vi "Get ChildType.vi"(8 "error in (no error)":errorcluster, 11 "LVArrayType.lvclass in":refnum<class "LVArrayType.lvclass">) -> (0 "error out":errorcluster, 2 "ChildType":refnum<class "LVType.lvclass">, 3 "LVArrayType.lvclass out":refnum<class "LVArrayType.lvclass">)   [LabVIEW 2020, in "LVDataTypes.lvlib" / "LVArrayType.lvclass"]
uses:
  <vilib>/AppBuilder/Engine/WebServiceDescription/LVDataTypes/LVArrayType/LVArrayType.lvclass
  <vilib>/AppBuilder/Engine/WebServiceDescription/LVDataTypes/LVType/LVType.lvclass
  <vilib>/AppBuilder/Engine/WebServiceDescription/LVDataTypes/LVArrayType/LVArrayType.lvclass/LVArrayType.ctl
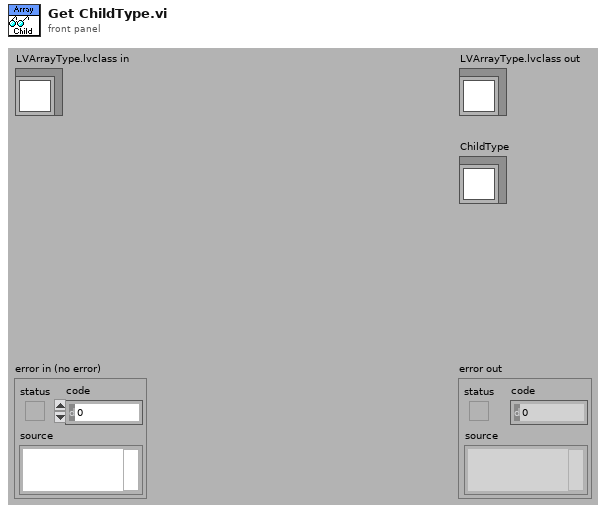
[diagram p1: front panel]
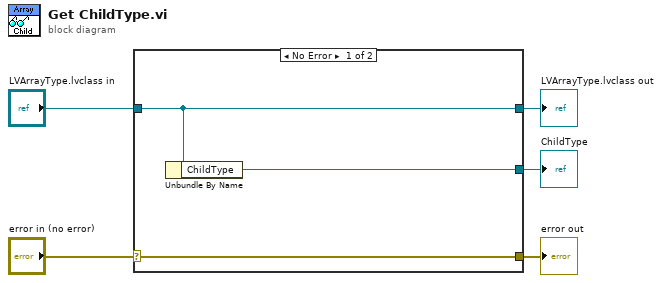
[diagram p0: block diagram]
diagram:
  n1 = case shown="No Error" "error in (no error)" {
    selector: "error in (no error)" -> [w8 w9]
    tunnel: [w8 w9] -> w4
    tunnel: [w7 w10] -> w2
    tunnel: "LVArrayType.lvclass in" -> [w7 w10]
    tunnel: [w6 _] -> w1
    frame No Error {
      n2 = Unbundle By Name(w7) -> ("ChildType"=w6:refnum<class "LVType.lvclass">)
    }
    frame Error {
    }
  }
  "error out" <- w4
  "LVArrayType.lvclass out" <- w2
  "ChildType" <- w1
